vi "Status.vi"(8 "error in (no error)":errorcluster, 11 "Response Msg in":refnum<class "Response Msg.lvclass">) -> (0 "error out":errorcluster, 1 "Time to Timeout (ms)":i32, 2 "Dropped?":bool, 3 "Response Msg out":refnum<class "Response Msg.lvclass">)   [LabVIEW 2020, in "Publisher.lvlib" / "Response Msg.lvclass"]
doc: "Check if the Response Core has been dropped. A dropped core indicates an interrupt or timeout state which should lead to a termination of the Response Msg."
uses:
  Response Msg.lvclass
  Response Msg.lvclass/Response Msg.ctl
  Response Core/Response Core/Response Core.lvclass
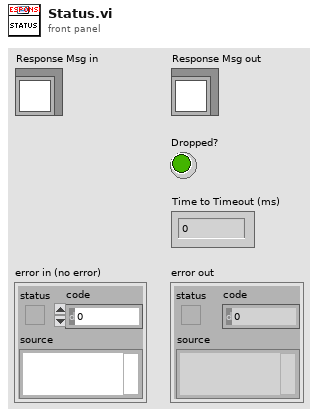
[diagram p1: front panel]
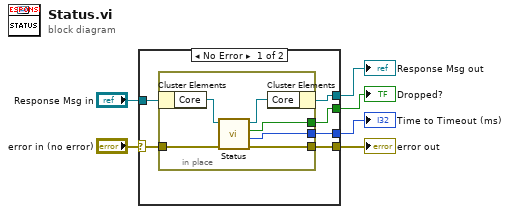
[diagram p0: block diagram]
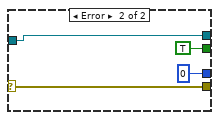
[diagram p2: hidden frame]
diagram:
  n1 = case shown="No Error" "error in (no error)" {
    selector: "error in (no error)" -> [w9 w22]
    tunnel: "Response Msg in" -> [w12 w20]
    tunnel: [w11 w20] -> w5
    tunnel: [w8 w22] -> w3
    tunnel: [w10 TRUE ("Timeout?")] -> w2
    tunnel: [w7 0 ("Time to Timeout (ms)")] -> w1
    frame No Error {
      n2 = in-place {
        in-place-border: [w16] -> w10
        in-place-border: w9 -> [w15]
        in-place-border: [w14] -> w8
        in-place-border: [w13] -> w7
        n3 = in-place-cluster #1(w12) -> ("Core"=w18:refnum<class "Response Core.lvclass">)
        n4 = call-dynamic "Status.vi"("error in (no error)"=w15, "Response Core in"=w18) -> ("error out"=w14:errorcluster, "Time to Timeout (ms)"=w13:i32, "Dropped?"=w16:bool, "Response Core out"=w17:refnum<class "Response Core.lvclass">)  [unwired: 6 in]
        n5 = in-place-cluster #1("Core"=w17) -> (w11:refnum<class "Response Msg.lvclass">)
      }
    }
    frame Error {
    }
  }
  "error out" <- w3
  "Response Msg out" <- w5
  "Dropped?" <- w2
  "Time to Timeout (ms)" <- w1
